vi "ERR HANDLER - Stop Loop.vi"(8 "error in":errorcluster) -> (0 "error out":errorcluster)   [LabVIEW 2013]
uses:
  Error Queue Message.ctl
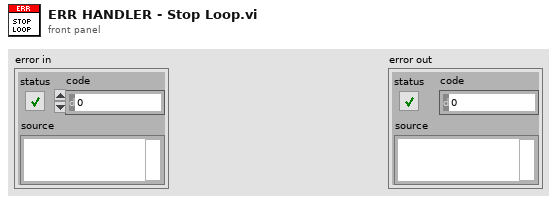
[diagram p1: front panel]
types:
  T1 = typedef "Error Queue Message.ctl" = cluster{"Command":enum16{"HANDLE ERROR", "EXIT"}, "Data":variant}
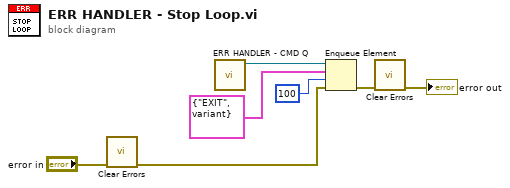
[diagram p0: block diagram]
diagram:
  n1 = call <vilib>:"Clear Errors.vi"("error in (no error)"="error in") -> ("error out"=w4:errorcluster)  [unwired: 6 in]
  n2 = call "ERR HANDLER - CMD Q.vi"() -> ("Err Handler Q"=w7:refnum<queue>)  [unwired: 11 in]
  n3 = Enqueue Element(queue=w7, element=T1 {"Command"=enum."EXIT", "Data"=variant} ("Error Handler Mesg"), timeout in ms (-1)=100, error in (no error)=w4) -> (error out=w3:errorcluster)  [unwired: 2 out]
  n4 = call <vilib>:"Clear Errors.vi"("error in (no error)"=w3) -> ("error out"=→"error out":errorcluster)  [unwired: 6 in]
